vi "plot_wave_mat.vi"() -> ()   [LabVIEW 2016]
panel:
  out "subarray 3":string[][](array[string])
  out "subarray 2":string[][](array[string])
  in  "File Path Control":path
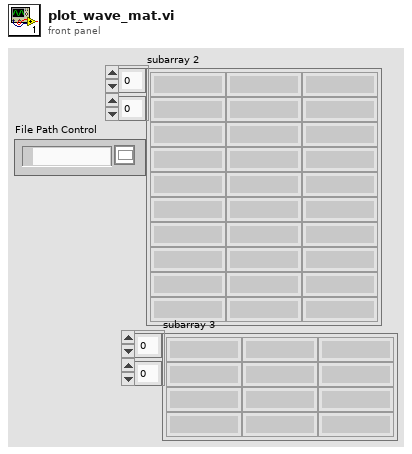
[diagram p1: front panel]
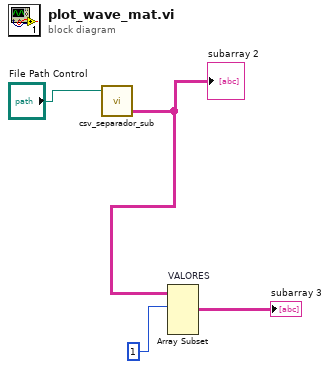
[diagram p0: block diagram]
diagram:
  n1 = call "csv_separador_sub.vi"("Archivo de referencias (.csv)"="File Path Control") -> ("subarray 2"=w1:string[][])  [unwired: 2 in, 2 out]
  "subarray 2" <- w1
  n2 = Array Subset "VALORES"(array=w1, index (row)=1 ("index")) -> (→"subarray 3":string[][])  [unwired: 3 in]
